vi "tsdiag_can_input_output_control_by_identifier.vi"(6 "data in":u8[](array[numeric]) format="%.0x", 7 "mode":u8(ring) items=["ReturnControlToECU", "ResetToDefault", "FreezeCurrentState", "ShortTermAdjustment"], 8 "error in (no error)":errorcluster, 9 "ID":u16 format="%.0x", 10 "ADiagModuleIndex":i32, 11 "path":path) -> (0 "error out":errorcluster, 1 "success?":bool, 2 "Return Type":i32, 3 "path out":path, 4 "data out":u8[](array[numeric]) format="%.0x")   [LabVIEW 2014]
doc: "2F服务，按标识符输入输出控制。"
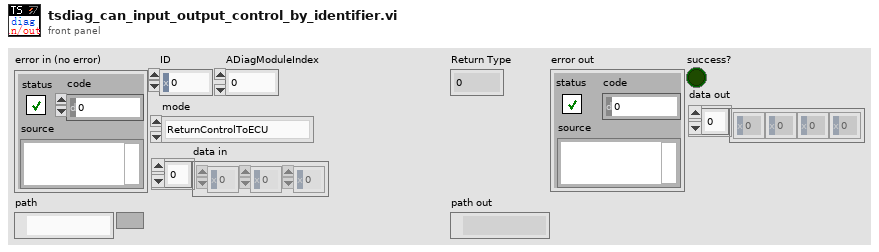
[diagram p1: front panel]
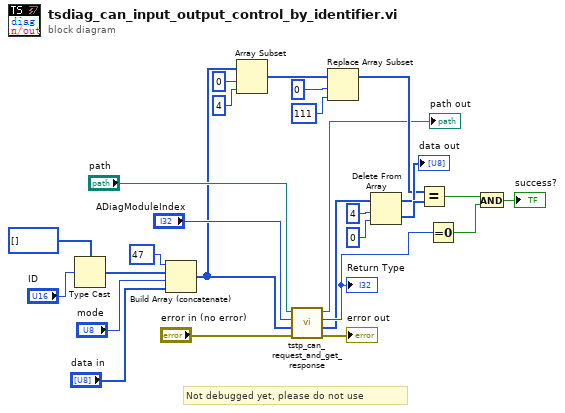
[diagram p0: block diagram]
diagram:
  # "Not debugged yet, please do not use"
  n1 = Type Cast(type=u8[] [], x="ID") -> (*(type *) &x=w12:u8[])
  n2 = Build Array (concatenate)(u8 47 ("element"), w12, "mode", "data in") -> (w4:u8[])
  n3 = Array Subset(array=w4, index=0, length=4) -> (w17:u8[])
  n4 = call "tstp_can_request_and_get_response.vi"("错误输入（无错误）"="error in (no error)", "AReqDataArray"=w4, "ADiagModuleIndex"="ADiagModuleIndex", "path"="path") -> ("错误输出"=→"error out":errorcluster, "Diagnostic response"=w1:u8[], "Return Type"=w3:i32, "path out"=→"path out":path)  [unwired: 4 in]
  "Return Type" <- w3
  n5 = Replace Array Subset(array=w17, new element=u8 111 ("new element/subarray"), index=0) -> (w14:u8[])
  n6 = Delete From Array(array=w1, length=4, index=0) -> (deleted portion=w24:u8[], array with subset deleted=→"data out":u8[])
  n7 = Equal?(x=w14, y=w24) -> (x = y?=w22:bool)
  n8 = Equal To 0?(x=w3) -> (x = 0?=w2:bool)
  n9 = And(x=w22, y=w2) -> (x .and. y?=→"success?":bool)
